vi "FIFOtoHost.vi"(7 "FIFO control":T5, 9 "Line Status In":T3, 11 "Data":T4={"Single Channel Output"={"Single Channel Data out"=0, "Output Valid"=FALSE, "Pixel Overwritten by Tag"=FALSE}, "Multi Channel Output"={"Multi Channel Data out"=[0, 0, 0, 0], "Output Valid"=FALSE, "Pixel Overwritten by Tag"=FALSE}}) -> (1 "FIFO Multi Channels Pixels Lost":u32, 2 "FIFO Single Channels Pixels Lost":u32, 3 "IRQ Flags Out":T1)   [LabVIEW 2014]
uses:
  Acquisition Engine/Acquisition Status.ctl
  IRQ/IRQ Flags.ctl
panel:
  # "Copyright 2014 Vidrio Technologies\nScanImage 5 software is licensed under the Apache License, Version 2.0 (the \"License\"); you may not use any files contained\nwithin the ScanImage 5 release except in compliance with the License. You may obtain a copy of the License at\n http://www.apache.org/licenses/LICENSE-2.0\nUnless required by applicable law or agreed to in writing, software distributed under the License is distributed on an\n\"AS IS\" BASIS, WITHOUT WARRANTIES OR CONDITIONS OF ANY KIND, either express or implied. See the License for the\n specific language governing permissions and limitations under the License."
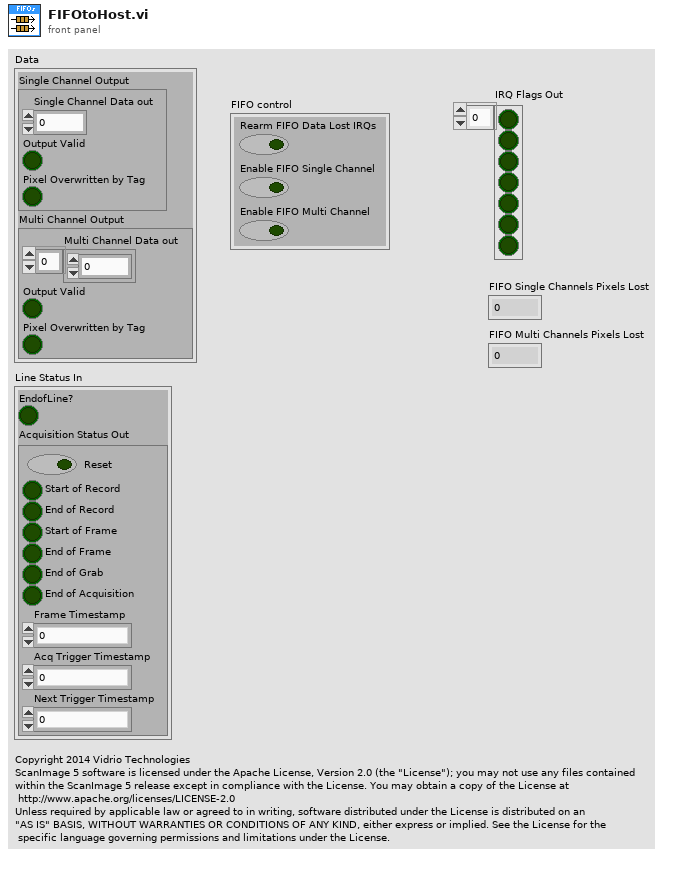
[diagram p1: front panel]
types:
  T1 = typedef "IRQ Flags.ctl" = bool[]
  T2 = typedef "Acquisition Status.ctl" = cluster{"Reset":bool, "Start of Record":bool, "End of Record":bool, "Start of Frame":bool, "End of Frame":bool, "End of Grab":bool, "End of Acquisition":bool, "Frame Timestamp":u64, "Acq Trigger Timestamp":u64, "Next Trigger Timestamp":u64}
  T3 = cluster{"EndofLine?":bool, "Acquisition Status Out":T2}
  T4 = cluster{"Single Channel Output":cluster{"Single Channel Data out":i16, "Output Valid":bool, "Pixel Overwritten by Tag":bool}, "Multi Channel Output":cluster{"Multi Channel Data out":i16[], "Output Valid":bool, "Pixel Overwritten by Tag":bool}}
  T5 = cluster{"Rearm FIFO Data Lost IRQs":bool, "Enable FIFO Single Channel":bool, "Enable FIFO Multi Channel":bool}
  T6 = cluster{"Single Channel Data out":i16, "Output Valid":bool, "Pixel Overwritten by Tag":bool}
  T7 = cluster{"Multi Channel Data out":i16[], "Output Valid":bool, "Pixel Overwritten by Tag":bool}
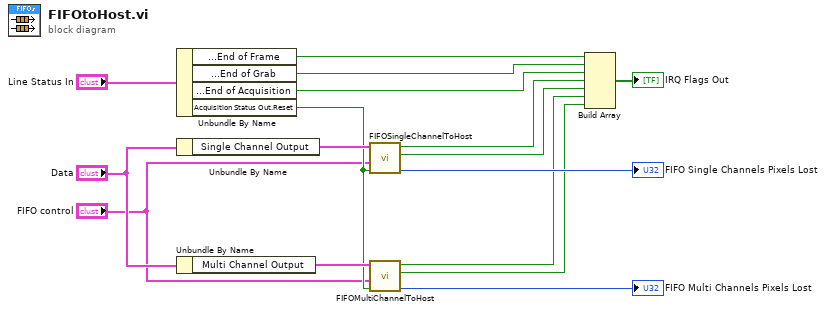
[diagram p0: block diagram]
diagram:
  n1 = Unbundle By Name("Line Status In") -> ("Acquisition Status Out.End of Frame"=w11:bool, "Acquisition Status Out.End of Grab"=w10:bool, "Acquisition Status Out.End of Acquisition"=w9:bool, "Acquisition Status Out.Reset"=w8:bool)
  n2 = Unbundle By Name("Data") -> ("Single Channel Output"=w16:T6)
  n3 = Unbundle By Name("Data") -> ("Multi Channel Output"=w14:T7)
  n4 = call "FIFOSingleChannelToHost.vi"("Reset"=w8, "FIFO control"="FIFO control", "Single Channel"=w16) -> ("FIFO Single Channels Pixels Lost"=→"FIFO Single Channels Pixels Lost":u32, "assert pixel overwritten interrupt"=w4:bool, "assert FIFO overflow interrupt"=w13:bool)  [unwired: 6 in]
  n5 = call "FIFOMultiChannelToHost.vi"("Reset"=w8, "FIFO control"="FIFO control", "Multi Channel Data"=w14) -> ("FIFO Multi Channels Pixels Lost"=→"FIFO Multi Channels Pixels Lost":u32, "assert pixel overwritten interrupt"=w2:bool, "assert FIFO overflow interrupt"=w3:bool)  [unwired: 6 in]
  n6 = Build Array(w11, w10, w9, w13, w4, w3, w2) -> (→"IRQ Flags Out":bool[])
